vi "VI Tree.vi"   [LabVIEW 2018, in "Agilent U2000 Series.lvlib"]
doc: "This is the instrument driver for the Agilent U2000 series power sensor (U2000A/B/H, U2001A/B/H, U2002A/H and U2004A, U2021XA, U2022XA, U2041XA, U2042XA, U2043XA, U2044XA, U2049XA). The VI Tree displays all the user-callable VIs of the instrument driver in an organized table."
uses:
  Agilent U2000 Series.lvlib
  Data/Read CCDF (Trace).vi
  Data/Low Level/Initiate (Immediate).vi
panel:
  # "(c) 2011-2015 National Instruments.  ALL RIGHTS RESERVED."
  # "SEE DIAGRAM\nFOR VI TREE."
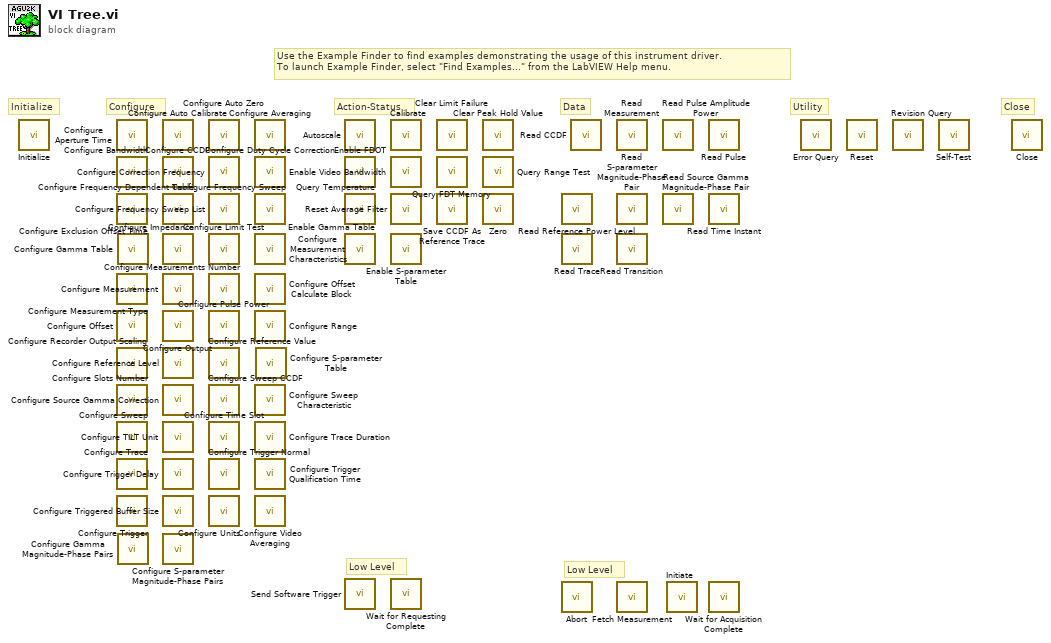
[diagram p0: block diagram]
diagram:
  # "Low Level"
  # "Action-Status"
  # "Close"
  # "Utility"
  # "Low Level"
  # "Data"
  # "Configure"
  # "Initialize"
  # "Use the Example Finder to find examples demonstrating the usage of this instrument driver.\nTo launch Example Finder, select \"Find Examples...\" from the LabVIEW Help menu."
  n1 = call "Initialize.vi"() -> ()  [unwired: 10 in, 2 out]
  n2 = call "Configure Aperture Time.vi"() -> ()  [unwired: 10 in, 2 out]
  n3 = call "Configure Bandwidth.vi"() -> ()  [unwired: 10 in, 2 out]
  n4 = call "Configure Exclusion Offset Time.vi"() -> ()  [unwired: 10 in, 2 out]
  n5 = call "Configure Measurement Type.vi"() -> ()  [unwired: 10 in, 2 out]
  n6 = call "Configure Offset.vi"() -> ()  [unwired: 10 in, 2 out]
  n7 = call "Configure Recorder Output Scaling.vi"() -> ()  [unwired: 10 in, 2 out]
  n8 = call "Configure Slots Number.vi"() -> ()  [unwired: 10 in, 2 out]
  n9 = call "Configure Sweep.vi"() -> ()  [unwired: 10 in, 2 out]
  n10 = call "Configure Trace.vi"() -> ()  [unwired: 10 in, 2 out]
  n11 = call "Configure Trigger.vi"() -> ()  [unwired: 14 in, 2 out]
  n12 = call "Configure Gamma Table.vi"() -> ()  [unwired: 10 in, 2 out]
  n13 = call "Configure Gamma Magnitude-Phase Pairs.vi"() -> ()  [unwired: 10 in, 2 out]
  n14 = call "Configure Auto Calibrate.vi"() -> ()  [unwired: 10 in, 2 out]
  n15 = call "Configure CCDF.vi"() -> ()  [unwired: 10 in, 2 out]
  n16 = call "Configure Frequency Dependent Table.vi"() -> ()  [unwired: 10 in, 2 out]
  n17 = call "Configure Impedance.vi"() -> ()  [unwired: 10 in, 2 out]
  n18 = call "Configure Measurement.vi"() -> ()  [unwired: 10 in, 2 out]
  n19 = call "Configure Output.vi"() -> ()  [unwired: 10 in, 2 out]
  n20 = call "Configure Reference Level.vi"() -> ()  [unwired: 10 in, 2 out]
  n21 = call "Configure Source Gamma Correction.vi"() -> ()  [unwired: 10 in, 2 out]
  n22 = call "Configure TILT Unit.vi"() -> ()  [unwired: 10 in, 2 out]
  n23 = call "Configure Trigger Delay.vi"() -> ()  [unwired: 10 in, 2 out]
  n24 = call "Configure Triggered Buffer Size.vi"() -> ()  [unwired: 10 in, 2 out]
  n25 = call "Configure S-parameter Magnitude-Phase Pairs.vi"() -> ()  [unwired: 10 in, 2 out]
  n26 = call "Configure Auto Zero.vi"() -> ()  [unwired: 10 in, 2 out]
  n27 = call "Configure Correction Frequency.vi"() -> ()  [unwired: 10 in, 2 out]
  n28 = call "Configure Frequency Sweep List .vi"() -> ()  [unwired: 10 in, 2 out]
  n29 = call "Configure Limit Test.vi"() -> ()  [unwired: 10 in, 2 out]
  n30 = call "Configure Measurements Number.vi"() -> ()  [unwired: 10 in, 2 out]
  n31 = call "Configure Pulse Power.vi"() -> ()  [unwired: 10 in, 2 out]
  n32 = call "Configure Reference Value.vi"() -> ()  [unwired: 10 in, 2 out]
  n33 = call "Configure Sweep CCDF.vi"() -> ()  [unwired: 10 in, 2 out]
  n34 = call "Configure Time Slot.vi"() -> ()  [unwired: 10 in, 2 out]
  n35 = call "Configure Trigger Normal.vi"() -> ()  [unwired: 10 in, 2 out]
  n36 = call "Configure Units.vi"() -> ()  [unwired: 10 in, 2 out]
  n37 = call "Configure Averaging.vi"() -> ()  [unwired: 10 in, 2 out]
  n38 = call "Configure Duty Cycle Correction.vi"() -> ()  [unwired: 10 in, 2 out]
  n39 = call "Configure Frequency Sweep.vi"() -> ()  [unwired: 10 in, 2 out]
  n40 = call "Configure Measurement Characteristics.vi"() -> ()  [unwired: 14 in, 2 out]
  n41 = call "Configure Offset Calculate Block.vi"() -> ()  [unwired: 10 in, 2 out]
  n42 = call "Configure Range.vi"() -> ()  [unwired: 10 in, 2 out]
  n43 = call "Configure Sweep Characteristic.vi"() -> ()  [unwired: 10 in, 2 out]
  n44 = call "Configure Trace Duration.vi"() -> ()  [unwired: 10 in, 2 out]
  n45 = call "Configure Trigger Qualification Time.vi"() -> ()  [unwired: 10 in, 2 out]
  n46 = call "Configure Video Averaging.vi"() -> ()  [unwired: 10 in, 2 out]
  n47 = call "Configure S-parameter Table.vi"() -> ()  [unwired: 10 in, 2 out]
  n48 = call "Autoscale.vi"() -> ()  [unwired: 10 in, 2 out]
  n49 = call "Enable FDOT.vi"() -> ()  [unwired: 10 in, 2 out]
  n50 = call "Query Temperature.vi"() -> ()  [unwired: 9 in, 3 out]
  n51 = call "Enable Gamma Table.vi"() -> ()  [unwired: 10 in, 2 out]
  n52 = call "Send Software Trigger.vi"() -> ()  [unwired: 10 in, 2 out]
  n53 = call "Calibrate.vi"() -> ()  [unwired: 9 in, 3 out]
  n54 = call "Enable Video Bandwidth.vi"() -> ()  [unwired: 10 in, 2 out]
  n55 = call "Reset Average Filter.vi"() -> ()  [unwired: 10 in, 2 out]
  n56 = call "Enable S-parameter Table.vi"() -> ()  [unwired: 10 in, 2 out]
  n57 = call "Wait for Requesting Complete.vi"() -> ()  [unwired: 10 in, 2 out]
  n58 = call "Clear Limit Failure.vi"() -> ()  [unwired: 10 in, 2 out]
  n59 = call "Query FDT Memory.vi"() -> ()  [unwired: 11 in, 5 out]
  n60 = call "Save CCDF As Reference Trace.vi"() -> ()  [unwired: 10 in, 2 out]
  n61 = call "Clear Peak Hold Value.vi"() -> ()  [unwired: 10 in, 2 out]
  n62 = call "Query Range Test.vi"() -> ()  [unwired: 8 in, 4 out]
  n63 = call "Zero.vi"() -> ()  [unwired: 10 in, 2 out]
  n64 = call "Read Reference Power Level.vi"() -> ()  [unwired: 9 in, 3 out]
  n65 = call "Read Trace.vi"() -> ()  [unwired: 9 in, 3 out]
  n66 = call "Abort.vi"() -> ()  [unwired: 10 in, 2 out]
  n67 = call-poly "Read CCDF.vi"() -> ()  [unwired: 7 in, 5 out]
  n68 = call "Read Measurement.vi"() -> ()  [unwired: 9 in, 3 out]
  n69 = call "Read S-parameter Magnitude-Phase Pair.vi"() -> ()  [unwired: 8 in, 4 out]
  n70 = call "Read Transition.vi"() -> ()  [unwired: 6 in, 6 out]
  n71 = call "Fetch Measurement.vi"() -> ()  [unwired: 9 in, 3 out]
  n72 = call "Read Pulse Amplitude Power.vi"() -> ()  [unwired: 7 in, 5 out]
  n73 = call "Read Source Gamma Magnitude-Phase Pair.vi"() -> ()  [unwired: 8 in, 4 out]
  n74 = call-poly "Initiate.vi"() -> ()  [unwired: 10 in, 2 out]
  n75 = call "Read Pulse.vi"() -> ()  [unwired: 6 in, 6 out]
  n76 = call "Read Time Instant.vi"() -> ()  [unwired: 8 in, 4 out]
  n77 = call "Wait for Acquisition Complete.vi"() -> ()  [unwired: 10 in, 2 out]
  n78 = call "Error Query.vi"() -> ()  [unwired: 8 in, 4 out]
  n79 = call "Reset.vi"() -> ()  [unwired: 10 in, 2 out]
  n80 = call "Revision Query.vi"() -> ()  [unwired: 8 in, 4 out]
  n81 = call "Self-Test.vi"() -> ()  [unwired: 8 in, 4 out]
  n82 = call "Close.vi"() -> ()  [unwired: 11 in, 1 out]
